vi "Read Benchmarks.vi"(8 "error in (no error)":errorcluster, 11 "CIFCorePlugin in":refnum<class "CIFCorePlugin.lvclass">) -> (0 "error out":errorcluster, 2 "Benchmarks":T1, 3 "CIFCorePlugin out":refnum<class "CIFCorePlugin.lvclass">)   [LabVIEW 2021, in "CIFCorePlugin.lvclass"]
uses:
  CIFCorePlugin.lvclass
  CIFCorePlugin.lvclass/CIFCorePlugin.ctl
  <vilib>/CIF Foundation/CIF Utilities/Statistics/I64/Stats_I64_CIF_U.lvclass
  Typedef/Benchmarks.ctl
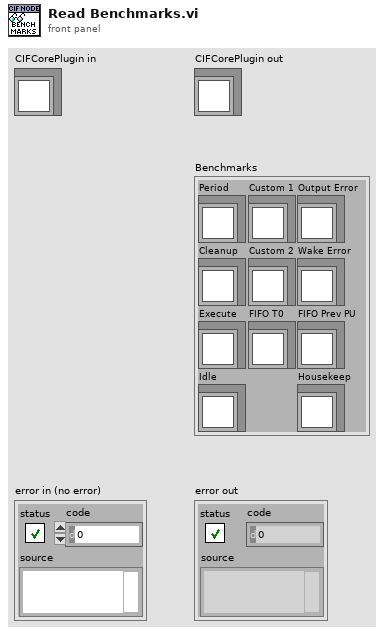
[diagram p1: front panel]
types:
  T1 = typedef "CIFCorePlugin.lvclass/Benchmarks.ctl" = cluster{"Period":refnum<class "Stats_I64_CIF_U.lvclass">, "Wake Error":refnum<class "Stats_I64_CIF_U.lvclass">, "Execute":refnum<class "Stats_I64_CIF_U.lvclass">, "Housekeep":refnum<class "Stats_I64_CIF_U.lvclass">, "Idle":refnum<class "Stats_I64_CIF_U.lvclass">, "Cleanup":refnum<class "Stats_I64_CIF_U.lvclass">, "FIFO T0":refnum<class "Stats_I64_CIF_U.lvclass">, "FIFO Prev PU":refnum<class "Stats_I64_CIF_U.lvclass">, "Output Error":refnum<class "Stats_I64_CIF_U.lvclass">, "Custom 1":refnum<class "Stats_I64_CIF_U.lvclass">, "Custom 2":refnum<class "Stats_I64_CIF_U.lvclass">}
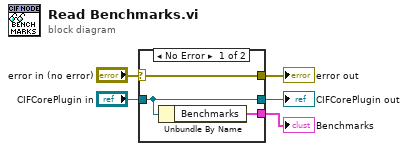
[diagram p0: block diagram]
diagram:
  n1 = case shown="No Error" "error in (no error)" {
    selector: "error in (no error)" -> [w8 w9]
    tunnel: [w8 w9] -> w4
    tunnel: [w7 w10] -> w2
    tunnel: "CIFCorePlugin in" -> [w7 w10]
    tunnel: [w6 _] -> w1
    frame No Error {
      n2 = Unbundle By Name(w7) -> ("Benchmarks"=w6:T1)
    }
    frame Error {
    }
  }
  "error out" <- w4
  "CIFCorePlugin out" <- w2
  "Benchmarks" <- w1
